vi "23384_Davis_Poku_Amankwa_Amankwa.DavisPoku.MNE1201.5.1_348259_1393773701.vi"() -> ()   [LabVIEW 2018]
panel:
  out "array":dbl[][](array[numeric])
  out "text":string
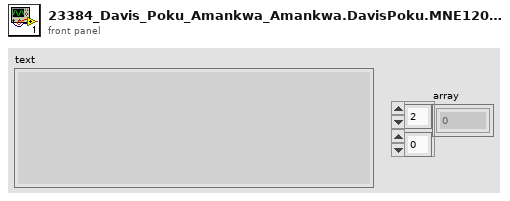
[diagram p1: front panel]
types:
  T1 = enum16{"open", "replace", "create", "open or create", "replace or create", "replace or create with confirmation"}
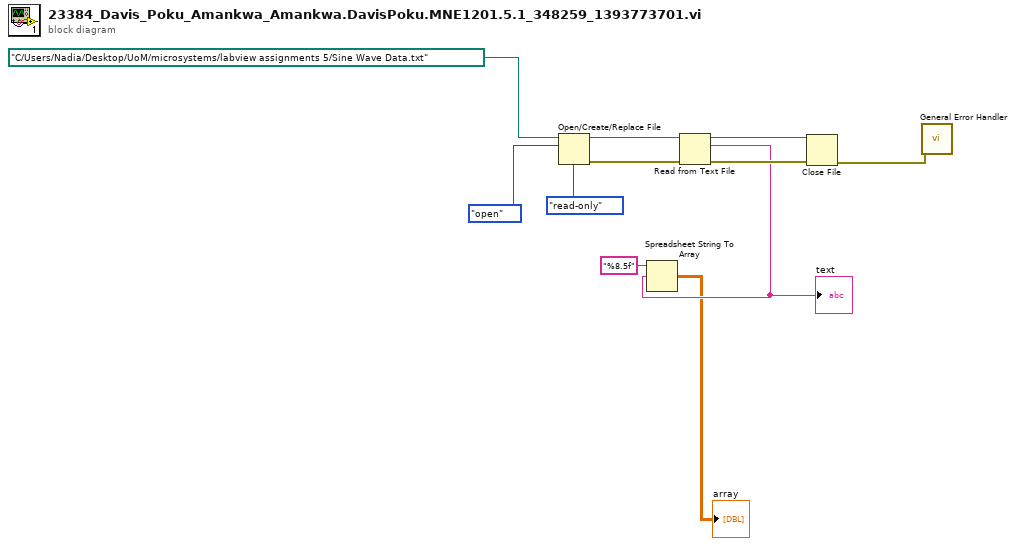
[diagram p0: block diagram]
diagram:
  n1 = Open/Create/Replace File(file path (use dialog)=path "C:/Users/Nadia/Desktop/UoM/microsystems/labview assignments 5/Sine Wave Data.txt", operation (0:open)=T1."open", access (0:read/write)=enum16{"read/write", "read-only", "write-only"}."read-only") -> (refnum out=w9:refnum<file>, error out=w8:errorcluster)  [unwired: 3 in, 1 out]
  n2 = Read from Text File(file (use dialog)=w9, error in=w8) -> (refnum out=w7:refnum<file>, text=w3:string, error out=w6:errorcluster)  [unwired: 2 in, 1 out]
  "text" <- w3
  n3 = Spreadsheet String To Array(format string="%8.5f", spreadsheet string=w3) -> (array=→"array":dbl[][])  [unwired: 2 in]
  n4 = Close File(refnum=w7, error in=w6) -> (error out=w5:errorcluster)  [unwired: 1 out]
  n5 = call <vilib>:"General Error Handler.vi"("error in (no error)"=w5) -> ()  [unwired: 10 in, 5 out]
